vi "TrajectoryParam_timeParam.vi"(9 "TRAJECTORY_CONFIG":T1={"MaxVelocity"=0.0, "Max Acceleration"=0.0, "StartVelocity"=0.0, "End Velocity"=0.0, "Reversed"=FALSE, "DiffDrKineConstntDefined"=FALSE, "CentAcellConstntDefined"=FALSE, "DiffDrVoltConstntDefined"=FALSE, "DIFF_DRIVE_KINE_CONSTRAINT"={"Max Speed (M/S)"=0.0, "DIFF_DRIVE_KINEMATICS"={"TrackWidth_Meters"=0.0}}, "CENTRIPETAL_ACCEL_CONSTRAINT"={"Max Cent Accel"=0.0}, "SwerveDrKineConstntDefined"=FALSE, "SWERVE_DRIVE_KINE_CONSTRAINT"={"Max Speed (M/S)"=0.0, "SwerveKinematics"={"NumModules"=0, "InverseKinematics"=[], "ForwardKinematics"=[], "Modules"=[], "PrevCoR"={"X"=0.0, "Y"=0.0}}}, "DIFF_DRIVE_VOLTAGE_CONSTRAINT"={"Max Voltage"=0.0, "DIFF_DRIVE_KINEMATICS"={"TrackWidth_Meters"=0.0}, "SIMPLE_MOTOR_FF"={"Ks"=0.0, "Kv"=0.0, "Ka"=0.0}}, "MECANUM_DRIVE_KINE_CONSTRAINT"={"Max Speed (M/S)"=0.0, "MECA_DRIVE_KINEMATICS"={"FrontLeft"={"X"=0.0, "Y"=0.0}, "FrontRight"={"X"=0.0, "Y"=0.0}, "RearLeft"={"X"=0.0, "Y"=0.0}, "RearRight"={"X"=0.0, "Y"=0.0}, "InverseKinematics"=[[0.0, 1.0, -1.0, 0.0], [0.0, 1.0, 1.0, 0.0], [0.0, 1.0, 1.0, 0.0], [0.0, 1.0, -1.0, 0.0]], "ForwardKinematics"=[[0.0, 1.0, -1.0, 0.0], [0.0, 1.0, 1.0, 0.0], [0.0, 1.0, 1.0, 0.0], [0.0, 1.0, -1.0, 0.0]], "PrevCoR"={"X"=0.0, "Y"=0.0}}}, "MecanumDrKineConstntDefined"=FALSE} {"MECANUM_DRIVE_KINE_CONSTRAINT"."MECA_DRIVE_KINEMATICS"."PrevCoR"."Y" format="%14.3f"; "MECANUM_DRIVE_KINE_CONSTRAINT"."MECA_DRIVE_KINEMATICS"."PrevCoR"."X" format="%14.3f"; "MECANUM_DRIVE_KINE_CONSTRAINT"."MECA_DRIVE_KINEMATICS"."RearRight"."Y" format="%14.3f"; "MECANUM_DRIVE_KINE_CONSTRAINT"."MECA_DRIVE_KINEMATICS"."RearRight"."X" format="%14.3f"; "MECANUM_DRIVE_KINE_CONSTRAINT"."MECA_DRIVE_KINEMATICS"."RearLeft"."Y" format="%14.3f"; "MECANUM_DRIVE_KINE_CONSTRAINT"."MECA_DRIVE_KINEMATICS"."RearLeft"."X" format="%14.3f"; "MECANUM_DRIVE_KINE_CONSTRAINT"."MECA_DRIVE_KINEMATICS"."FrontRight"."Y" format="%14.3f"; "MECANUM_DRIVE_KINE_CONSTRAINT"."MECA_DRIVE_KINEMATICS"."FrontRight"."X" format="%14.3f"; "MECANUM_DRIVE_KINE_CONSTRAINT"."MECA_DRIVE_KINEMATICS"."FrontLeft"."Y" format="%14.3f"; "MECANUM_DRIVE_KINE_CONSTRAINT"."MECA_DRIVE_KINEMATICS"."FrontLeft"."X" format="%14.3f"; "MECANUM_DRIVE_KINE_CONSTRAINT"."Max Speed (M/S)" format="%20.4f"; "DIFF_DRIVE_VOLTAGE_CONSTRAINT"."SIMPLE_MOTOR_FF"."Ka" format="%13.4f"; "DIFF_DRIVE_VOLTAGE_CONSTRAINT"."SIMPLE_MOTOR_FF"."Kv" format="%13.4f"; "DIFF_DRIVE_VOLTAGE_CONSTRAINT"."SIMPLE_MOTOR_FF"."Ks" format="%13.4f"; "DIFF_DRIVE_VOLTAGE_CONSTRAINT"."DIFF_DRIVE_KINEMATICS"."TrackWidth_Meters" format="%20.4f"; "DIFF_DRIVE_VOLTAGE_CONSTRAINT"."Max Voltage" format="%20.4f"; "SWERVE_DRIVE_KINE_CONSTRAINT"."SwerveKinematics"."PrevCoR"."Y" format="%14.3f"; "SWERVE_DRIVE_KINE_CONSTRAINT"."SwerveKinematics"."PrevCoR"."X" format="%14.3f"; "SWERVE_DRIVE_KINE_CONSTRAINT"."SwerveKinematics"."Modules"."Y" format="%14.3f"; "SWERVE_DRIVE_KINE_CONSTRAINT"."SwerveKinematics"."Modules"."X" format="%14.3f"; "SWERVE_DRIVE_KINE_CONSTRAINT"."Max Speed (M/S)" format="%20.4f"; "CENTRIPETAL_ACCEL_CONSTRAINT"."Max Cent Accel" format="%20.4f"; "DIFF_DRIVE_KINE_CONSTRAINT"."DIFF_DRIVE_KINEMATICS"."TrackWidth_Meters" format="%20.4f"; "DIFF_DRIVE_KINE_CONSTRAINT"."Max Speed (M/S)" format="%20.4f"; "End Velocity" format="%20.4f"; "StartVelocity" format="%20.4f"; "Max Acceleration" format="%20.4f"; "MaxVelocity" format="%20.4f"}, 11 "points":T17[](array[typedef]) {"POSE"."ROTATION"."SIN" format="%13.4f"; "POSE"."ROTATION"."COS" format="%13.4f"; "POSE"."ROTATION"."VALUE" format="%13.4f"; "POSE"."TRANSLATION"."Y" format="%14.3f"; "POSE"."TRANSLATION"."X" format="%14.3f"}) -> (0 "error out":errorcluster, 3 "TRAJECTORY":T13 {"States"."POSE"."ROTATION"."SIN" format="%13.4f"; "States"."POSE"."ROTATION"."COS" format="%13.4f"; "States"."POSE"."ROTATION"."VALUE" format="%13.4f"; "States"."POSE"."TRANSLATION"."Y" format="%14.3f"; "States"."POSE"."TRANSLATION"."X" format="%14.3f"; "TotalTImeSecs" format="%20.3f"})   [LabVIEW 2019, in "Trajectory_Library.lvlib"]
doc: "Parameterize the trajectory by time. This is where the velocity profile is generated.\n \nThe derivation of the algorithm used can be found here \"http://www2.informatik.uni-freiburg.de/~lau/students/Sprunk2008.pdf\"\n \n - points - The spline points.\n - TrajectoryConfig - Trajectory Config data structure (it contains - start velocity, end velocity, max velocity, max acceration, reversed, and constraint data)\n\nReturns:\n - Trajectory - Trajectory data structure\n - Error Out - Returned error cluster"
uses:
  Trajectory_Library.lvlib
  POSEwCURVATURE.ctl
  POSE2D.ctl
  TRANSLATION2D.ctl
  ROTATION2D.ctl
  TRAJECTORY.ctl
  TRAJ_STATE.ctl
  TRAJ_CONFIG.ctl
  TRAJ_CONSTRAINT_DIIF_DRIVE_KINEMATICS.ctl
  DIFF_DRIVE_KINEMATICS.ctl
  TRAJ_CONSTRAINT_CENTRIPETAL_ACCEL.ctl
  TRAJ_CONSTRAINT_SWERVE_DRIVE_KINEMATICS.ctl
  SWERVE_DRIVE_KINEMATICS.ctl
  <vilib>/Analysis/Matrix/Datatypes/RealMatrix.ctl
  TRAJ_CONSTRAINT_DIIF_DRIVE_VOLTAGE.ctl
  SIMPLE_MOTOR_FF.ctl
  TRAJ_CONSTRAINT_MECA_DRIVE_KINEMATICS.ctl
  MECA_DRIVE_KINEMATICS.ctl
  CONSTRAINED_STATE.ctl
  Util_CalcDist.vi
  <vilib>/Analysis/Matrix/NI_Matrix.lvlib
panel:
  # "ARRAY OF OTHER\nCONSTRAINTS \nGOES HERE.."
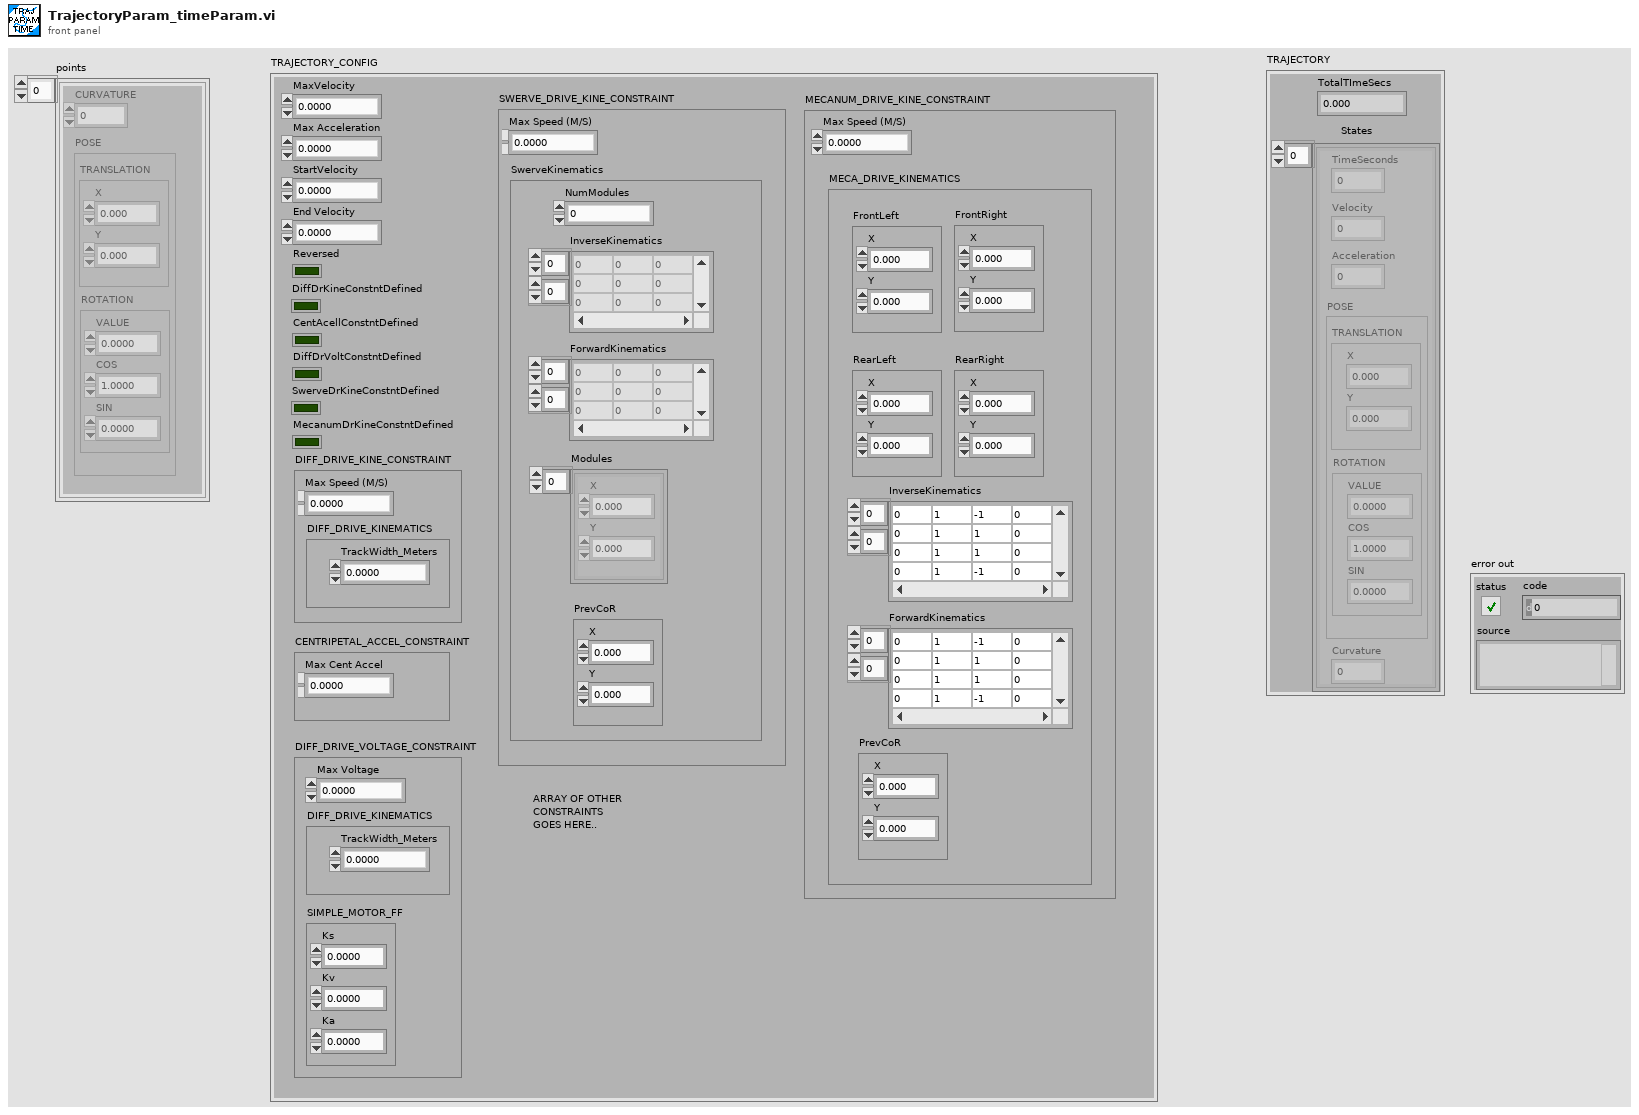
[diagram p1: front panel]
types:
  T1 = typedef "Trajectory_Library.lvlib/TRAJ_CONFIG.ctl" = cluster{"MaxVelocity":dbl, "Max Acceleration":dbl, "StartVelocity":dbl, "End Velocity":dbl, "Reversed":bool, "DiffDrKineConstntDefined":bool, "CentAcellConstntDefined":bool, "DiffDrVoltConstntDefined":bool, "DIFF_DRIVE_KINE_CONSTRAINT":T2, "CENTRIPETAL_ACCEL_CONSTRAINT":T4, "SwerveDrKineConstntDefined":bool, "SWERVE_DRIVE_KINE_CONSTRAINT":T5, "DIFF_DRIVE_VOLTAGE_CONSTRAINT":T9, "MECANUM_DRIVE_KINE_CONSTRAINT":T11, "MecanumDrKineConstntDefined":bool}
  T2 = typedef "Trajectory_Library.lvlib/TRAJ_CONSTRAINT_DIIF_DRIVE_KINEMATICS.ctl" = cluster{"Max Speed (M/S)":dbl, "DIFF_DRIVE_KINEMATICS":T3}
  T3 = typedef "Trajectory_Library.lvlib/DIFF_DRIVE_KINEMATICS.ctl" = cluster{"TrackWidth_Meters":dbl}
  T4 = typedef "Trajectory_Library.lvlib/TRAJ_CONSTRAINT_CENTRIPETAL_ACCEL.ctl" = cluster{"Max Cent Accel":dbl}
  T5 = typedef "Trajectory_Library.lvlib/TRAJ_CONSTRAINT_SWERVE_DRIVE_KINEMATICS.ctl" = cluster{"Max Speed (M/S)":dbl, "SwerveKinematics":T6}
  T6 = typedef "Trajectory_Library.lvlib/SWERVE_DRIVE_KINEMATICS.ctl" = cluster{"NumModules":i32, "InverseKinematics":T7, "ForwardKinematics":T7, "Modules":T8[], "PrevCoR":T8}
  T7 = typedef "NI_Matrix.lvlib/RealMatrix.ctl" = dbl[][]
  T8 = typedef "Trajectory_Library.lvlib/TRANSLATION2D.ctl" = cluster{"X":dbl, "Y":dbl}
  T9 = typedef "Trajectory_Library.lvlib/TRAJ_CONSTRAINT_DIIF_DRIVE_VOLTAGE.ctl" = cluster{"Max Voltage":dbl, "DIFF_DRIVE_KINEMATICS":T3, "SIMPLE_MOTOR_FF":T10}
  T10 = typedef "Trajectory_Library.lvlib/SIMPLE_MOTOR_FF.ctl" = cluster{"Ks":dbl, "Kv":dbl, "Ka":dbl}
  T11 = typedef "Trajectory_Library.lvlib/TRAJ_CONSTRAINT_MECA_DRIVE_KINEMATICS.ctl" = cluster{"Max Speed (M/S)":dbl, "MECA_DRIVE_KINEMATICS":T12}
  T12 = typedef "Trajectory_Library.lvlib/MECA_DRIVE_KINEMATICS.ctl" = cluster{"FrontLeft":T8, "FrontRight":T8, "RearLeft":T8, "RearRight":T8, "InverseKinematics":T7, "ForwardKinematics":T7, "PrevCoR":T8}
  T13 = typedef "Trajectory_Library.lvlib/TRAJECTORY.ctl" = cluster{"TotalTImeSecs":dbl, "States":T14[]}
  T14 = typedef "Trajectory_Library.lvlib/TRAJ_STATE.ctl" = cluster{"TimeSeconds":dbl, "Velocity":dbl, "Acceleration":dbl, "POSE":T15, "Curvature":dbl}
  T15 = typedef "Trajectory_Library.lvlib/POSE2D.ctl" = cluster{"TRANSLATION":T8, "ROTATION":T16}
  T16 = typedef "Trajectory_Library.lvlib/ROTATION2D.ctl" = cluster{"VALUE":dbl, "COS":dbl, "SIN":dbl}
  T17 = typedef "Trajectory_Library.lvlib/POSEwCURVATURE.ctl" = cluster{"CURVATURE":dbl, "POSE":T15}
  T18 = typedef "Trajectory_Library.lvlib/CONSTRAINED_STATE.ctl" = cluster{"POSEwCURVATURE":T17, "Distance":dbl, "minAccel":dbl, "maxAccel":dbl, "maxVelocity":dbl}
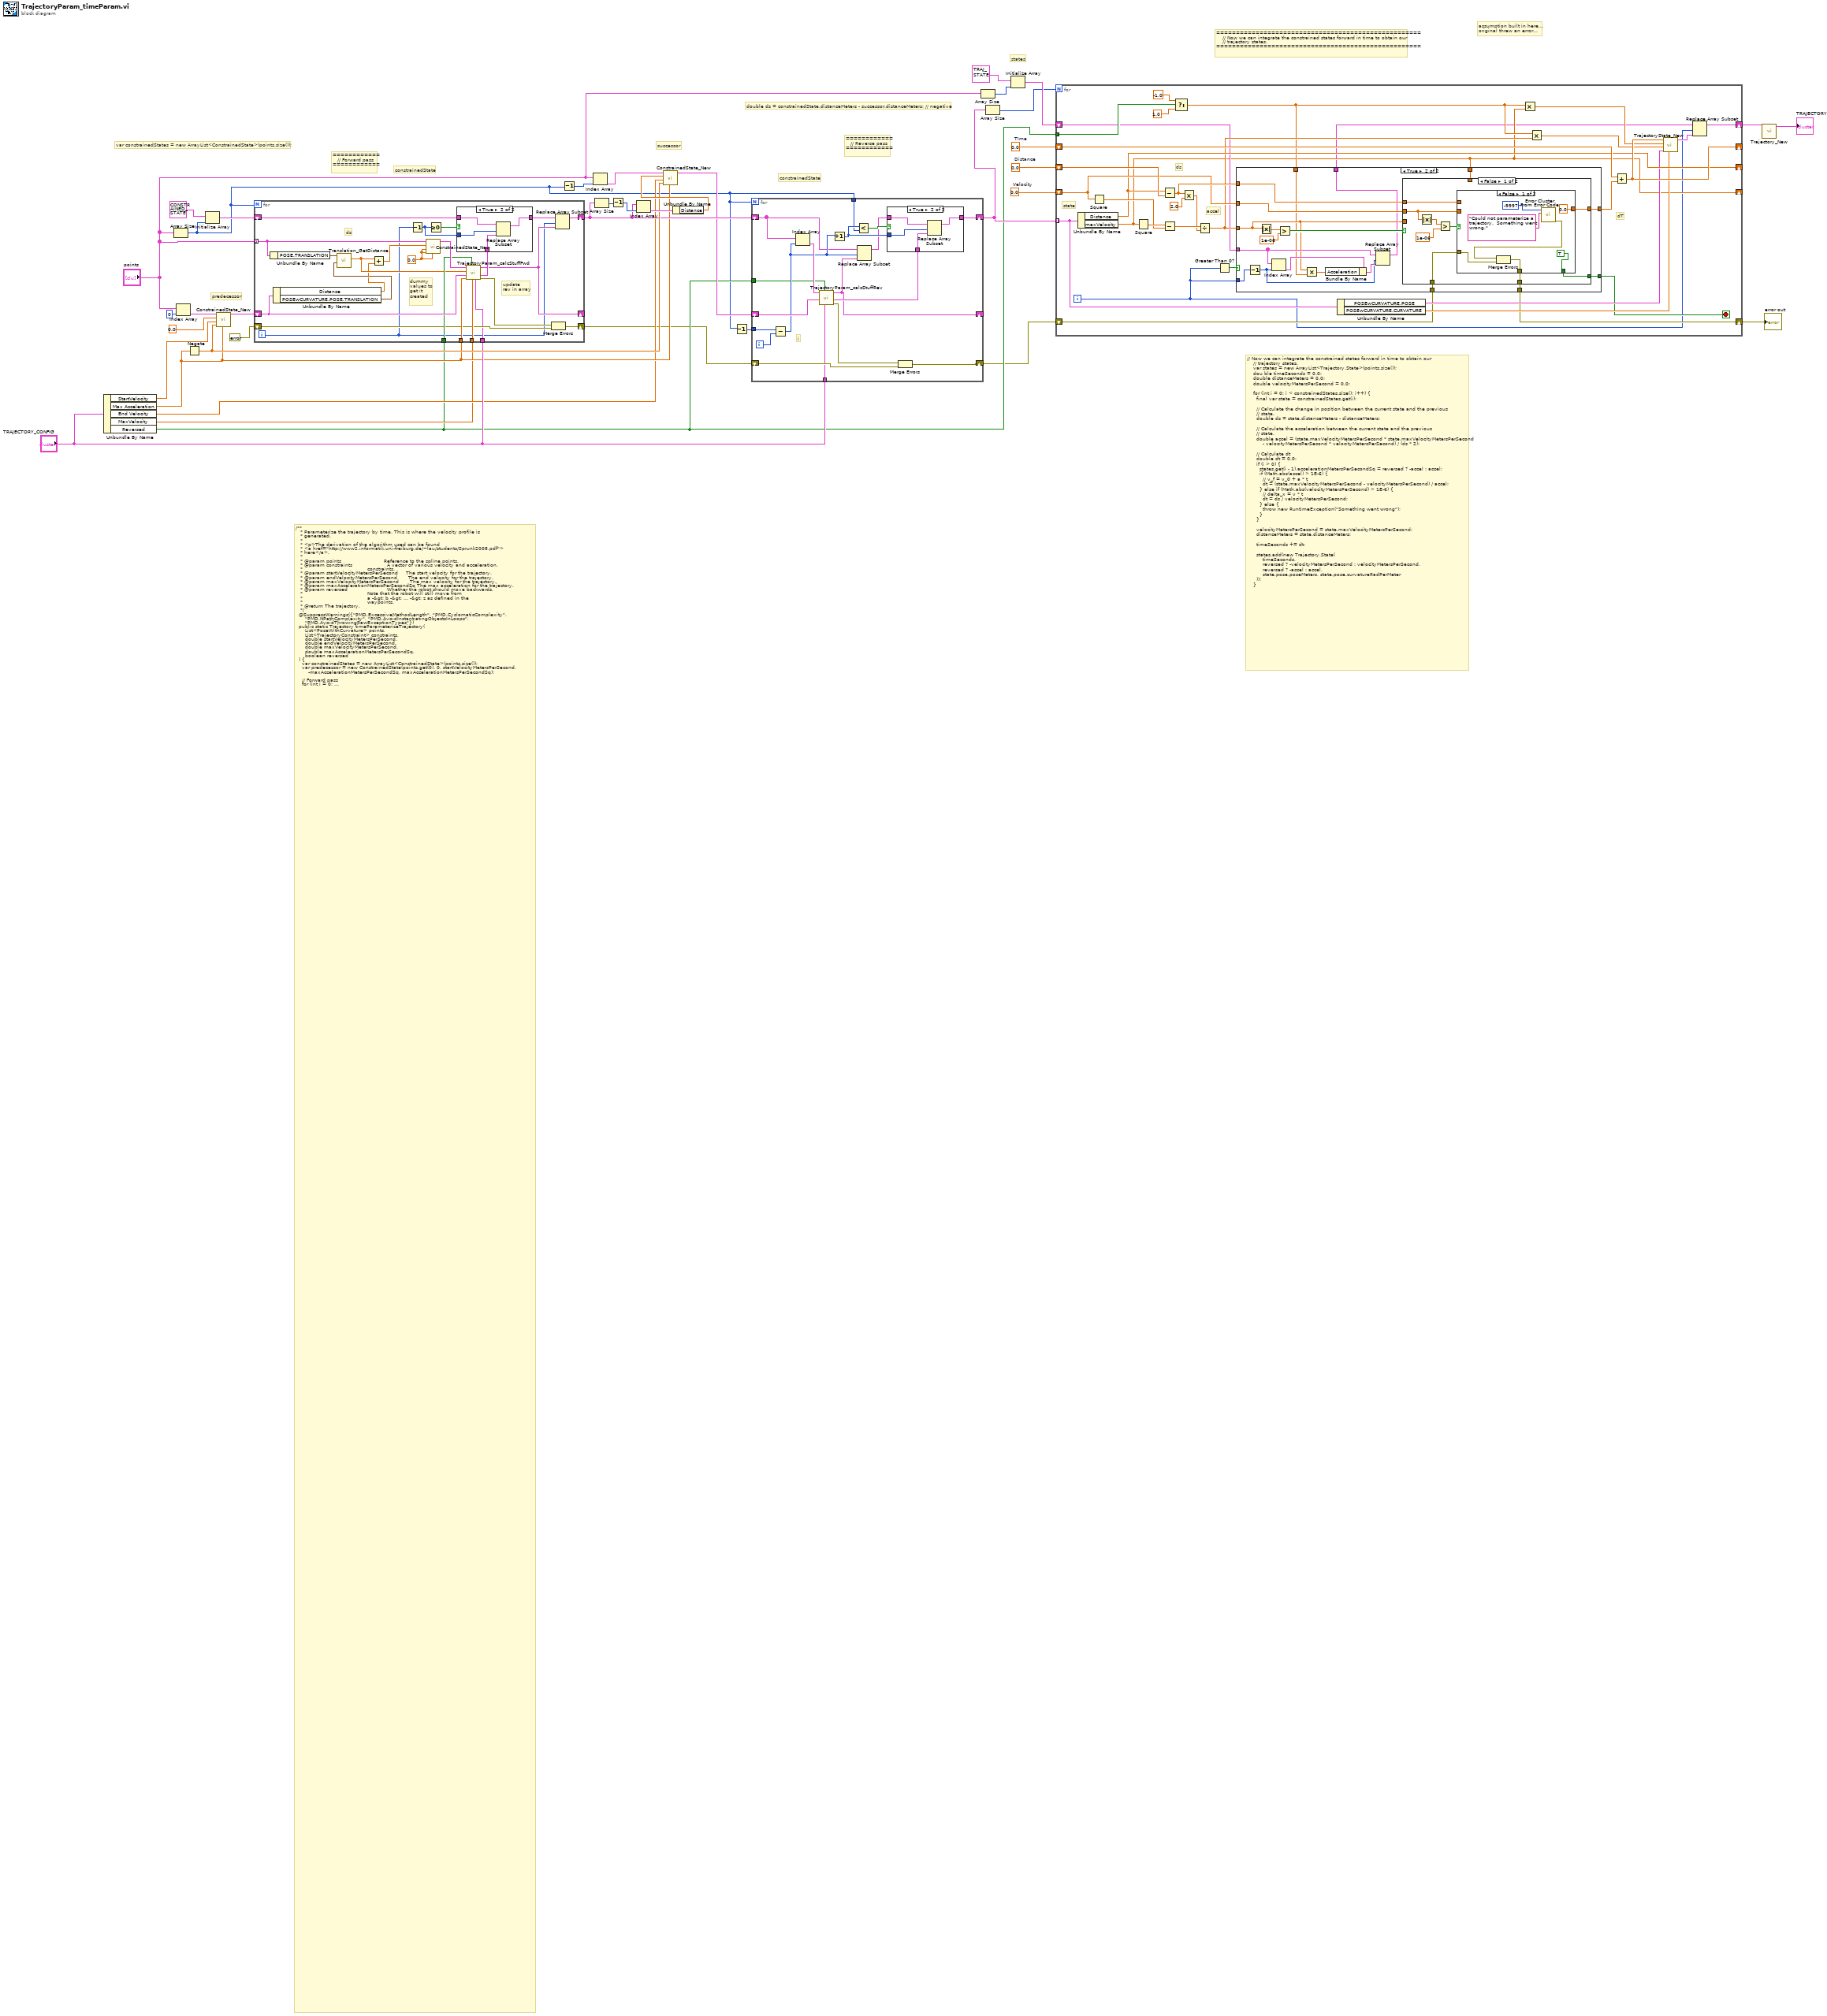
[diagram p0: block diagram]
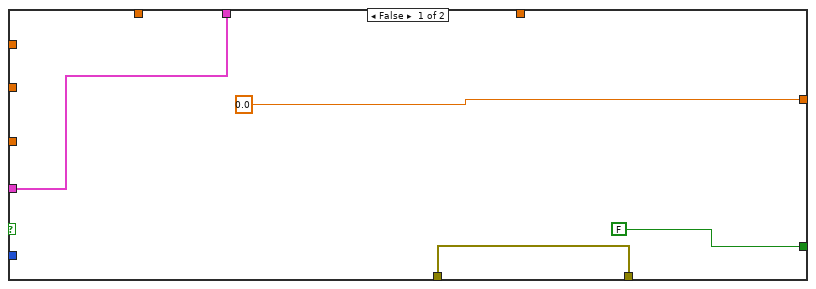
[diagram p2: hidden frame]
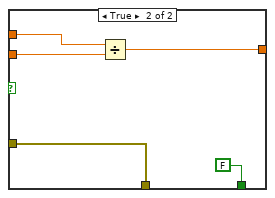
[diagram p3: hidden frame]
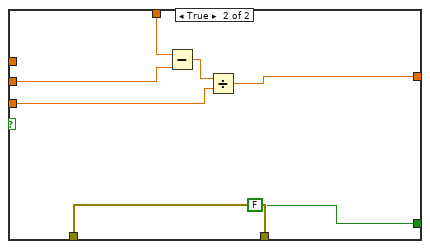
[diagram p4: hidden frame]
diagram:
  w20 = 0.0  # Velocity
  w21 = 0.0  # Distance
  w22 = 0.0  # TIme
  # "assumption built in here...\noriginal threw an error..."
  # "states"
  # "====================================================\n    // Now we can integrate the constrained states forward in time to obtain our\n    // trajectory states.\n===================================================="
  # "============\n   // Reverse pass\n============"
  # "constrainedState"
  # "// Now we can integrate the constrained states forward in time to obtain our\n    // trajectory states.\n    var states = new ArrayList<Trajectory.State>(points.size());\n    dou ble timeSeconds = 0.0;\n    double distanceMeters = 0.0;\n    double velocityMetersPerSecond = 0.0;\n\n    for (int i = 0; i < constrainedStates.size(); i++) {\n      final var state = constrainedStates.get(i);\n\n      // Calculate the change in position between the current state and the previous\n      // state.\n      double ds = state.distanceMeters - distanceMeters;\n\n      // Calculate the acceleration between the current state and the previous\n      // state.\n      double accel = (state.maxVelocityMetersPerSecond * state.maxVelocityMetersPerSecond\n          - velocityMetersPerSecond * velocityMetersPerSecond) / (ds * 2);\n\n      // Calculate dt\n      double dt = 0.0;\n      if (i > 0) {\n        states.get(i - 1).accelerationMetersPerSecondSq = reversed ? -accel : accel;\n        if (Math.abs(accel) > 1E-6) {\n          // v_f = v_0 + a * t\n          dt = (state.maxVelocityMetersPerSecond - velocityMetersPerSecond) / accel;\n        } else if (Math.abs(velocityMetersPerSecond) > 1E-6) {\n          // delta_x = v * t\n          dt = ds / velocityMetersPerSecond;\n        } else {\n          throw new RuntimeException(\"Something went wrong\");\n        }\n      }\n\n      velocityMetersPerSecond = state.maxVelocityMetersPerSecond;\n      distanceMeters = state.distanceMeters;\n\n      timeSeconds += dt;\n\n      states.add(new Trajectory.State(\n          timeSeconds,\n          reversed ? -velocityMetersPerSecond : velocityMetersPerSecond,\n          reversed ? -accel : accel,\n          state.pose.poseMeters, state.pose.curvatureRadPerMeter\n      ));\n    }"
  # "double ds = constrainedState.distanceMeters - successor.distanceMeters; // negative"
  # "constrainedState"
  # "successor"
  # "============\n   // Forward pass\n============"
  # "predecessor"
  # "var constrainedStates = new ArrayList<ConstrainedState>(points.size());"
  # "/**\n   * Parameterize the trajectory by time. This is where the velocity profile is\n   * generated.\n   *\n   * <p>The derivation of the algorithm used can be found\n   * <a href=\"http://www2.informatik.uni-freiburg.de/~lau/students/Sprunk2008.pdf\">\n   * here</a>.\n   *\n   * @param points                           Reference to the spline points.\n   * @param constraints                      A vector of various velocity and acceleration.\n   *                                         constraints.\n   * @param startVelocityMetersPerSecond     The start velocity for the trajectory.\n   * @param endVelocityMetersPerSecond       The end velocity for the trajectory.\n   * @param maxVelocityMetersPerSecond       The max velocity for the trajectory.\n   * @param maxAccelerationMetersPerSecondSq The max acceleration for the trajectory.\n   * @param reversed                         Whether the robot should move backwards.\n   *                                         Note that the robot will still move from\n   *                                         a -&gt; b -&gt; ... -&gt; z as defined in the\n   *                                         waypoints.\n   * @return The trajectory.\n   */\n  @SuppressWarnings({\"PMD.ExcessiveMethodLength\", \"PMD.CyclomaticComplexity\",\n      \"PMD.NPathComplexity\", \"PMD.AvoidInstantiatingObjectsInLoops\",\n      \"PMD.AvoidThrowingRawExceptionTypes\"})\n  public static Trajectory timeParameterizeTrajectory(\n      List<PoseWithCurvature> points,\n      List<TrajectoryConstraint> constraints,\n      double startVelocityMetersPerSecond,\n      double endVelocityMetersPerSecond,\n      double maxVelocityMetersPerSecond,\n      double maxAccelerationMetersPerSecondSq,\n      boolean reversed\n  ) {\n    var constrainedStates = new ArrayList<ConstrainedState>(points.size());\n    var predecessor = new ConstrainedState(points.get(0), 0, startVelocityMetersPerSecond,\n        -maxAccelerationMetersPerSecondSq, maxAccelerationMetersPerSecondSq);\n\n    // Forward pass\n    for (int i = 0; i < points.size(); i++) {\n      constrainedStates.add(new ConstrainedState());\n      var constrainedState = constrainedStates.get(i);\n      constrainedState.pose = points.get(i);\n\n      // Begin constraining based on predecessor.\n      double ds = constrainedState.pose.poseMeters.getTranslation().getDistance(\n          predecessor.pose.poseMeters.getTranslation());\n\n      constrainedState.distanceMeters = predecessor.distanceMeters + ds;\n\n      // We may need to iterate to find the maximum end velocity and common\n      // acceleration, since acceleration limits may be a function of velocity.\n      while (true) {\n        // Enforce global max velocity and max reachable velocity by global\n        // acceleration limit. vf = std::sqrt(vi^2 + 2*a*d).\n        constrainedState.maxVelocityMetersPerSecond = Math.min(\n            maxVelocityMetersPerSecond,\n            Math.sqrt(predecessor.maxVelocityMetersPerSecond\n                * predecessor.maxVelocityMetersPerSecond\n                + predecessor.maxAccelerationMetersPerSecondSq * ds * 2.0)\n        ); \n\n        constrainedState.minAccelerationMetersPerSecondSq = -maxAccelerationMetersPerSecondSq;\n        constrainedState.maxAccelerationMetersPerSecondSq = maxAccelerationMetersPerSecondSq;\n\n        // At this point, the constrained state is fully constructed apart from\n        // all the custom-defined user constraints.\n        for (final var constraint : constraints) {\n          constrainedState.maxVelocityMetersPerSecond = Math.min(\n              constrainedState.maxVelocityMetersPerSecond,\n              constraint.getMaxVelocityMetersPerSecond(\n                  constrainedState.pose.poseMeters, constrainedState.pose.curvatureRadPerMeter,\n                  constrainedState.maxVelocityMetersPerSecond)\n          );\n        }  //for\n\n        // Now enforce all acceleration limits.\n        enforceAccelerationLimits(reversed, constraints, constrainedState);\n\n        if (ds < 1E-6) {\n          break;   // end while loop\n        }\n\n        // If the actual acceleration for this state is higher than the max\n        // acceleration that we applied, then we need to reduce the max\n        // acceleration of the predecessor and try again.\n        double actualAcceleration = (constrainedState.maxVelocityMetersPerSecond\n            * constrainedState.maxVelocityMetersPerSecond\n            - predecessor.maxVelocityMetersPerSecond * predecessor.maxVelocityMetersPerSecond)\n            / (ds * 2.0);\n\n        // If we violate the max acceleration constraint, let's modify the\n        // predecessor.\n        if (constrainedState.maxAccelerationMetersPerSecondSq < actualAcceleration - 1E-6) {\n          predecessor.maxAccelerationMetersPerSecondSq\n              = constrainedState.maxAccelerationMetersPerSecondSq;\n        } else {\n          // Constrain the predecessor's max acceleration to the current\n          // acceleration.\n          if (actualAcceleration > predecessor.minAccelerationMetersPerSecondSq) {\n            predecessor.maxAccelerationMetersPerSecondSq = actualAcceleration;\n          }  //if\n          // If the actual acceleration is less than the predecessor's min\n          // acceleration, it will be repaired in the backward pass.\n          break;\n        } // if\n      }  // while\n      predecessor = constrainedState;\n    }  //for\n    // --------end forward pass\n    //------------------------------------------------------------------------------------------\n    var successor = new ConstrainedState(points.get(points.size() - 1),\n        constrainedStates.get(constrainedStates.size() - 1).distanceMeters,\n        endVelocityMetersPerSecond,\n        -maxAccelerationMetersPerSecondSq, maxAccelerationMetersPerSecondSq);\n\n    // ------------------------------------------------------------------------------------------\n    // --------start backwards pass.\n    // Backward pass\n    for (int i = points.size() - 1; i >= 0; i--) {\n      var constrainedState = constrainedStates.get(i);\n\n      double ds = constrainedState.distanceMeters - successor.distanceMeters; // negative\n\n      while (true) {\n        // Enforce max velocity limit (reverse)\n        // vf = std::sqrt(vi^2 + 2*a*d), where vi = successor.\n        double newMaxVelocity = Math.sqrt(\n                   successor.maxVelocityMetersPerSecond * successor.maxVelocityMetersPerSecond\n                   + successor.minAccelerationMetersPerSecondSq * ds * 2.0\n                   );\n\n        // No more limits to impose! This state can be finalized.\n        if (newMaxVelocity >= constrainedState.maxVelocityMetersPerSecond) {\n           break;\n        }\n\n        constrainedState.maxVelocityMetersPerSecond = newMaxVelocity;\n\n        // Check all acceleration constraints with the new max velocity.\n        enforceAccelerationLimits(reversed, constraints, constrainedState);\n\n        if (ds > -1E-6) {\n          break;\n        }\n\n        // If the actual acceleration for this state is lower than the min\n        // acceleration, then we need to lower the min acceleration of the\n        // successor and try again.\n        double actualAcceleration = (constrainedState.maxVelocityMetersPerSecond\n            * constrainedState.maxVelocityMetersPerSecond\n            - successor.maxVelocityMetersPerSecond * successor.maxVelocityMetersPerSecond)\n            / (ds * 2.0);\n\n        if (constrainedState.minAccelerationMetersPerSecondSq > actualAcceleration + 1E-6) {\n          successor.minAccelerationMetersPerSecondSq\n              = constrainedState.minAccelerationMetersPerSecondSq;\n        } else {\n          successor.minAccelerationMetersPerSecondSq = actualAcceleration;\n          break;\n        }\n      }  // WHILE END\n      successor = constrainedState;\n    }   // FOR END\n\n    //--------end of reverse path\n    //-----------------------------------------------------------------------------------\n\n    // Now we can integrate the constrained states forward in time to obtain our\n    // trajectory states.\n    var states = new ArrayList<Trajectory.State>(points.size());\n    dou  ble timeSeconds = 0.0;\n    dou      ble distanceMeters = 0.0;\n    double velocityMetersPerSecond = 0.0;\n\n    for (int i = 0; i < constrainedStates.size(); i++) {\n      final var state = constrainedStates.get(i);\n\n      // Calculate the change in position between the current state and the previous\n      // state.\n      double ds = state.distanceMeters - distanceMeters;\n\n      // Calculate the acceleration between the current state and the previous\n      // state.\n      double accel = (state.maxVelocityMetersPerSecond * state.maxVelocityMetersPerSecond\n          - velocityMetersPerSecond * velocityMetersPerSecond) / (ds * 2);\n\n      // Calculate dt\n      double dt = 0.0;\n      if (i > 0) {\n        states.get(i - 1).accelerationMetersPerSecondSq = reversed ? -accel : accel;\n        if (Math.abs(accel) > 1E-6) {\n          // v_f = v_0 + a * t\n          dt = (state.maxVelocityMetersPerSecond - velocityMetersPerSecond) / accel;\n        } else if (Math.abs(velocityMetersPerSecond) > 1E-6) {\n          // delta_x = v * t\n          dt = ds / velocityMetersPerSecond;\n        } else {\n          throw new RuntimeException(\"Something went wrong\");\n        }\n      }\n\n      velocityMetersPerSecond = state.maxVelocityMetersPerSecond;\n      distanceMeters = state.distanceMeters;\n\n      timeSeconds += dt;\n\n      states.add(new Trajectory.State(\n          timeSeconds,\n          reversed ? -velocityMetersPerSecond : velocityMetersPerSecond,\n          reversed ? -accel : accel,\n          state.pose.poseMeters, state.pose.curvatureRadPerMeter\n      ));\n    }\n\n    return new Trajectory(states);\n  }"
  n1 = Unbundle By Name("TRAJECTORY_CONFIG") -> ("StartVelocity"=w11:dbl, "Max Acceleration"=w10:dbl, "End Velocity"=w9:dbl, "MaxVelocity"=w8:dbl, "Reversed"=w7:bool)
  n2 = Array Size(array="points") -> (size(s)=w4:i32)
  n3 = Index Array(array="points", index=0) -> (element=w36:T17)
  n4 = Negate(x=w10) -> (-x=w27:dbl)
  n5 = Initialize Array(T18 {"POSEwCURVATURE"={"CURVATURE"=0.0, "POSE"={"TRANSLATION"={"X"=0.0, "Y"=0.0}, "ROTATION"={"VALUE"=0.0, "COS"=1.0, "SIN"=0.0}}}, "Distance"=0.0, "minAccel"=0.0, "maxAccel"=0.0, "maxVelocity"=0.0} ("CONSTRAINED_STATE"), w4) -> (w34:T18[])
  n6 = call "ConstrainedState_New.vi"("maxAcceleration"=w10, "minAcceleration"=w27, "maxVelocity"=w11, "Distance"=0.0, "POSEwCURVATURE"=w36) -> ("CONSTRAINED_STATE"=w33:T18)  [unwired: 6 in]
  n7 = for {
    N: w4 -> [_]
    shift-right: [w42] -> w25
    shift-left: w34 -> [w54]
    tunnel: "points" -> [w62] mode=indexing
    shift-right: [w41] -> _
    shift-left: w33 -> [w59]
    tunnel: w10 -> [w57]
    tunnel: w8 -> [w56]
    tunnel: w7 -> [w49]
    shift-right: [w48] -> w6
    shift-left: errorcluster {"status"=FALSE, "code"=0, "source"=""} ("error constant") -> [w46]
    tunnel: "TRAJECTORY_CONFIG" -> [w45]
    i -> [w39]
    w58 = 0.0 ("maxVelocity")
    # "ds"
    # "dummy\nvalues to\nget it \ncreated"
    # "update\nrev in array"
    n8 = Unbundle By Name(w62) -> ("POSE.TRANSLATION"=w61:T8)
    n9 = Unbundle By Name(w59) -> ("Distance"=w40:dbl, "POSEwCURVATURE.POSE.TRANSLATION"=w55:T8)
    n10 = call "Translation_GetDistance.vi"("other Translation"=w55, "In Translation"=w61) -> ("Distance"=w44:dbl)  [unwired: 9 in]
    n11 = Add(x=w44, y=w40) -> (x+y=w50:dbl)
    n12 = Decrement(x=w39) -> (x-1=w52:i32)
    n13 = call "ConstrainedState_New.vi"("maxAcceleration"=w58, "minAcceleration"=w58, "maxVelocity"=w58, "Distance"=w50, "POSEwCURVATURE"=w62) -> ("CONSTRAINED_STATE"=w60:T18)  [unwired: 6 in]
    n14 = Greater Or Equal To 0?(x=w52) -> (x >= 0?=w53:bool)
    n15 = call "TrajectoryParam_calcStuffFwd.vi"("TRAJECTORY_CONFIG"=w45, "MaxVelocity"=w56, "Reversed"=w49, "MaxAccel"=w57, "previousCONSTRAINED_STATEin"=w59, "ds"=w44, "thisCONSTRAINED_STATEin"=w60) -> ("error out"=w47:errorcluster, "previousCONSTRAINED_STATEout"=w51:T18, "thisCONSTRAINED_STATEout"=w41:T18)  [unwired: 2 in]
    n16 = case shown="True" w53 {
      tunnel: [w63 w65] -> w43
      tunnel: w54 -> [w63 w66]
      tunnel: w52 -> [_ w67]
      tunnel: w51 -> [_ w64]
      frame False {
      }
      frame True {
        n17 = Replace Array Subset(array=w66, new element=w64, index=w67) -> (w65:T18[])
      }
    }
    n18 = Merge Errors(w47, w46) -> (w48:errorcluster)
    n19 = Replace Array Subset(array=w43, new element=w41, index=w39) -> (w42:T18[])
  }
  n20 = Decrement(x=w4) -> (x-1=w32:i32)
  n21 = Index Array(array="points", index=w32) -> (element=w26:T17)
  n22 = Array Size(array=w25) -> (size(s)=w31:i32)
  n23 = Decrement(x=w31) -> (x-1=w30:i32)
  n24 = Index Array(array=w25, index=w30) -> (element=w29:T18)
  n25 = Unbundle By Name(w29) -> ("Distance"=w28:dbl)
  n26 = call "ConstrainedState_New.vi"("maxAcceleration"=w10, "minAcceleration"=w27, "maxVelocity"=w9, "Distance"=w28, "POSEwCURVATURE"=w26) -> ("CONSTRAINED_STATE"=w24:T18)  [unwired: 6 in]
  n27 = Decrement(x=w4) -> (x-1=w3:i32)
  n28 = for {
    N: w4 -> [_]
    shift-right: [w74] -> _
    shift-left: w24 -> [w83]
    shift-right: [w81] -> w17
    shift-left: w25 -> [w76]
    tunnel: w4 -> [w79]
    tunnel: w7 -> [w73]
    shift-right: [w72] -> w5
    shift-left: w6 -> [w70]
    tunnel: "TRAJECTORY_CONFIG" -> [w69]
    tunnel: w3 -> [w68]
    i -> [w85]
    # "i"
    n29 = Subtract(x=w68, y=w85) -> (x-y=w77:i32)
    n30 = Index Array(array=w76, index=w77) -> (element=w84:T18)
    n31 = call "TrajectoryParam_calcStuffRev.vi"("TRAJECTORY_CONFIG"=w69, "Reversed"=w73, "successorCONSTRAINED_STATEin"=w83, "thisCONSTRAINED_STATEin"=w84) -> ("error out"=w71:errorcluster, "successorCONSTRAINED_STATEout"=w82:T18, "thisCONSTRAINED_STATEout"=w74:T18)  [unwired: 5 in]
    n32 = Increment(x=w77) -> (x+1=w80:i32)
    n33 = Less?(x=w80, y=w79) -> (x < y?=w78:bool)
    n34 = Replace Array Subset(array=w76, new element=w74, index=w77) -> (w75:T18[])
    n35 = case shown="True" w78 {
      tunnel: [w86 w88] -> w81
      tunnel: w75 -> [w86 w89]
      tunnel: w80 -> [_ w90]
      tunnel: w82 -> [_ w87]
      frame False {
      }
      frame True {
        n36 = Replace Array Subset(array=w89, new element=w87, index=w90) -> (w88:T18[])
      }
    }
    n37 = Merge Errors(w71, w70) -> (w72:errorcluster)
  }
  n38 = Array Size(array="points") -> (size(s)=w2:i32)
  n39 = Array Size(array=w17) -> (size(s)=w18:i32)
  n40 = Initialize Array(T14 {"TimeSeconds"=0.0, "Velocity"=0.0, "Acceleration"=0.0, "POSE"={"TRANSLATION"={"X"=0.0, "Y"=0.0}, "ROTATION"={"VALUE"=0.0, "COS"=1.0, "SIN"=0.0}}, "Curvature"=0.0} ("TRAJ_STATE"), w2) -> (w19:T14[])
  n41 = for {
    N: w18 -> [_]
    shift-right: [w111] -> _
    shift-left: w22 -> [w112]
    shift-right: [w110] -> _
    shift-left: w21 -> [w122]
    shift-right: [w98] -> _
    shift-left: w20 -> [w114]
    shift-right: [w94] -> w15
    shift-left: w19 -> [w100]
    tunnel: w17 -> [w109] mode=indexing
    tunnel: w7 -> [w104]
    shift-right: [w97] -> w16
    shift-left: w5 -> [w96]
    i -> [w91]
    stop <- w95 stop-if-true
    # "state"
    # "dT"
    # "accel"
    # "ds"
    n42 = Unbundle By Name(w109) -> ("Distance"=w110:dbl, "maxVelocity"=w98:dbl)
    n43 = Square(x=w114) -> (x^2=w120:dbl)
    n44 = Square(x=w98) -> (x^2=w121:dbl)
    n45 = Subtract(x=w110, y=w122) -> (x-y=w115:dbl)
    n46 = Subtract(x=w121, y=w120) -> (x-y=w118:dbl)
    n47 = Select(t=-1.0, s=w104, f=1.0) -> (s? t:f=w99:dbl)
    n48 = Multiply(x=w115, y=2.0) -> (x*y=w117:dbl)
    n49 = Divide(x=w118, y=w117) -> (x/y=w102:dbl)
    n50 = Greater Than 0?(x=w91) -> (x > 0?=w116:bool)
    n51 = case shown="True" w116 {
      tunnel: w115 -> [_ w139]
      tunnel: [0.0 w140] -> w113
      tunnel: w91 -> [_ w145]
      tunnel: w100 -> [w125 w137]
      tunnel: w102 -> [_ w133]
      tunnel: w114 -> [_ w141]
      tunnel: [w125 w135] -> w93
      tunnel: w99 -> [_ w132]
      tunnel: w98 -> [_ w131]
      tunnel: [w124 w129] -> w97
      tunnel: w96 -> [w124 w128]
      tunnel: [FALSE w127] -> w95
      frame False {
      }
      frame True {
        n52 = Decrement(x=w145) -> (x-1=w130:i32)
        n53 = Absolute Value(x=w133) -> (abs(x)=w144:dbl)
        n54 = Index Array(array=w137, index=w130) -> (element=w138:T14)
        n55 = Greater?(x=w144, y=1e-06) -> (0:w142:bool)
        n56 = Multiply(x=w133, y=w132) -> (x*y=w134:dbl)
        n57 = Bundle By Name(cluster=w138, "Acceleration"=w134) -> (w136:T14)
        n58 = Replace Array Subset(array=w137, new element=w136, index=w130) -> (w135:T14[])
        n59 = case shown="False" w142 {
          tunnel: w141 -> [w151 w173]
          tunnel: w133 -> [_ w171]
          tunnel: [w153 w170] -> w140
          tunnel: w139 -> [w154 _]
          tunnel: w131 -> [_ w169]
          tunnel: [w147 w168] -> w129
          tunnel: w128 -> [w148 w168]
          tunnel: [w146 FALSE] -> w127
          frame False {
            n60 = Absolute Value(x=w151) -> (abs(x)=w152:dbl)
            n61 = Greater?(x=w152, y=1e-06) -> (0:w149:bool)
            n62 = case shown="False" w149 {
              tunnel: w154 -> [_ w166]
              tunnel: [0.0 w165] -> w153
              tunnel: w151 -> [_ w164]
              tunnel: w148 -> [w156 w163]
              tunnel: [w155 w163] -> w147
              tunnel: [TRUE FALSE] -> w146
              frame False {
                n63 = call <vilib>:"Error Cluster From Error Code.vi"("error message (\"\")"="Could not parameterize a trajectory.  Something went wrong." ("error message (\"\")"), "error code (0)"=-9997) -> ("error out"=w160:errorcluster)  [unwired: 7 in]
                n64 = Merge Errors(w160, w156) -> (w155:errorcluster)
              }
              frame True {
                n65 = Divide(x=w166, y=w164) -> (x/y=w165:dbl)
              }
            }
          }
          frame True {
            n66 = Subtract(x=w169, y=w173) -> (x-y=w172:dbl)
            n67 = Divide(x=w172, y=w171) -> (x/y=w170:dbl)
          }
        }
      }
    }
    n68 = Unbundle By Name(w109) -> ("POSEwCURVATURE.POSE"=w108:T15, "POSEwCURVATURE.CURVATURE"=w107:dbl)
    n69 = Multiply(x=w99, y=w98) -> (x*y=w103:dbl)
    n70 = Multiply(x=w99, y=w102) -> (x*y=w101:dbl)
    n71 = Add(x=w112, y=w113) -> (x+y=w111:dbl)
    n72 = call "TrajectoryState_New.vi"("Curvature"=w107, "POSE"=w108, "Accel"=w101, "Velocity"=w103, "Time"=w111) -> ("TRAJ_STATE"=w92:T14)  [unwired: 6 in]
    n73 = Replace Array Subset(array=w93, new element=w92, index=w91) -> (w94:T14[])
  }
  "error out" <- w16
  n74 = call "Trajectory_New.vi"("TRAJ_STATES"=w15) -> ("TRAJECTORY"=→"TRAJECTORY":T13)  [unwired: 10 in]
